vi "Data Rad For Buffer AI.vi"(8 "error In":errorcluster, 10 "Start Address":i32=1350, 11 "connection ID IN":refnum<k5>) -> (0 "error out":errorcluster, 2 "Data":dbl[](array[numeric]) format="%#.6f", 3 "connection ID OUT":refnum<k5>)   [LabVIEW 2015]
panel:
  out "concatenated string":string
  out "Array":string[](array[string])
  out "Numeric":i32
  out "bytes written1":i32
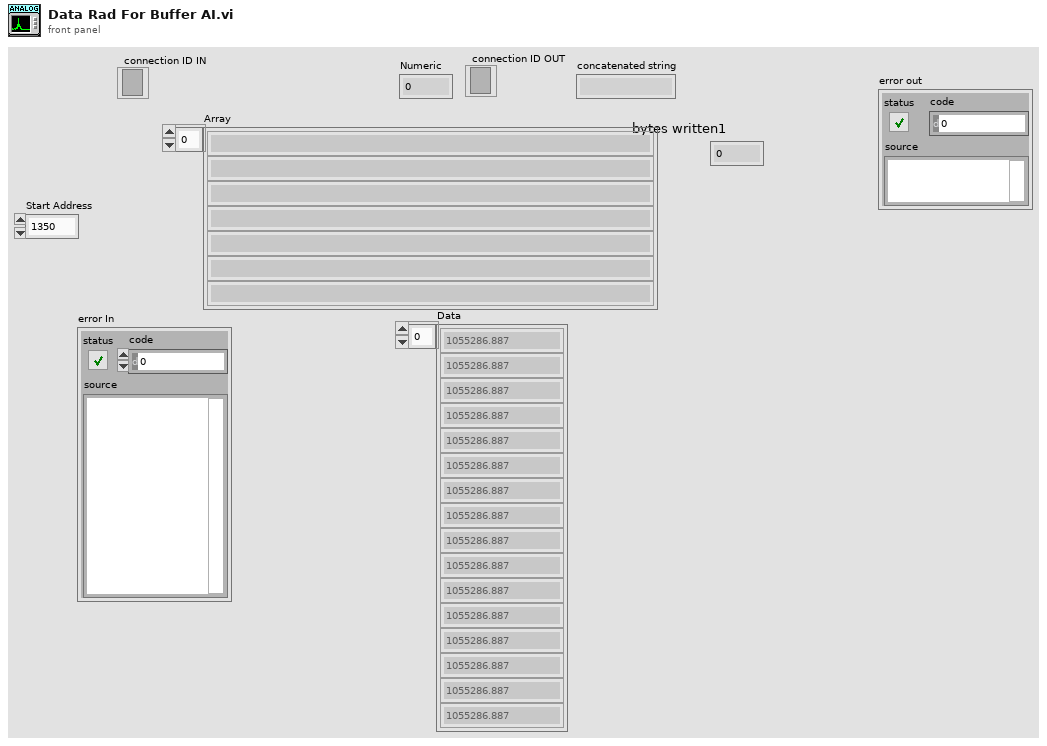
[diagram p1: front panel]
types:
  T1 = enum16{"Standard", "Buffered", "CRLF", "Immediate"}
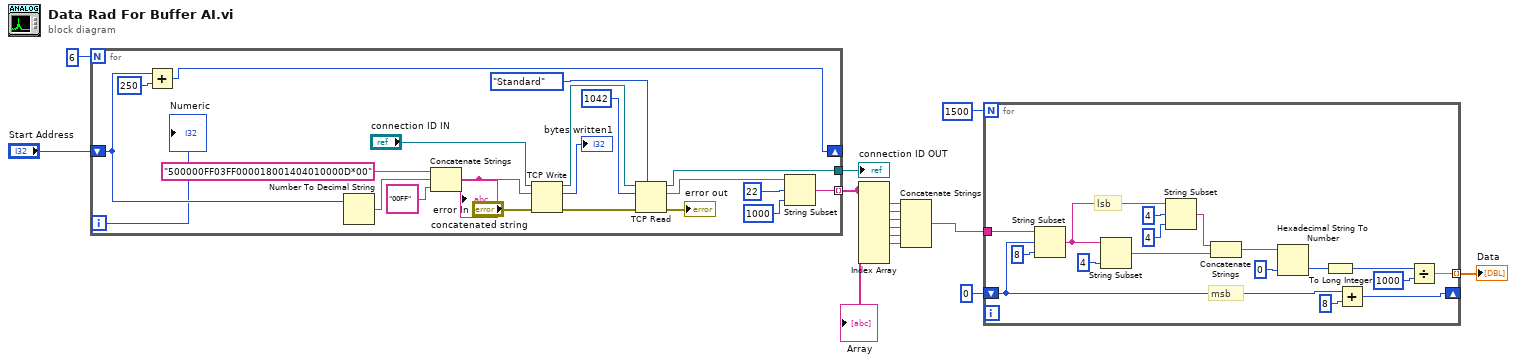
[diagram p0: block diagram]
diagram:
  n1 = for {
    N: 6 -> [_]
    tunnel: [w18] -> w9 mode=indexing
    tunnel: [w25] -> w13
    shift-right: [w22] -> _
    shift-left: "Start Address" -> [w24]
    i -> [w15]
    n2 = Add(x=w24, y=250) -> (x+y=w22:i32)
    n3 = Number To Decimal String(number=w24) -> (decimal integer string=w32:string)  [unwired: 1 in]
    n4 = Concatenate Strings("500000FF03FF000018001404010000D*00", w32, "00FF" ("String")) -> (w34:string)
    "concatenated string" <- w34
    n5 = TCP Write(connection ID="connection ID IN", data in=w34, error in (no error)="error In") -> (connection ID out=w29:refnum<k5>, bytes written=→"bytes written1":i32, error out=w28:errorcluster)  [unwired: 1 in]
    n6 = TCP Read(connection ID=w29, bytes to read=1042, error in (no error)=w28, 7:T1."Standard" ("mode (standard)")) -> (connection ID out=w25:refnum<k5>, data out=w19:string, error out=→"error out":errorcluster)  [unwired: 1 in]
    n7 = String Subset(string=w19, offset (0)=22, length (rest)=1000 ("length (rest)")) -> (substring=w18:string)
    "Numeric" <- w15
  }
  "connection ID OUT" <- w13
  "Array" <- w9
  n8 = Index Array(array=w9) -> (element #1=w7:string, element #2=w6:string, element #3=w5:string, element #4=w4:string, element #5=w2:string, element #6=w1:string)  [unwired: 8 in, 2 out]
  n9 = Concatenate Strings(w7, w6, w5, w4, w2, w1) -> (w3:string)
  n10 = for {
    N: 1500 ("Length") -> [_]
    shift-right: [w52] -> _
    shift-left: 0 -> [w49]
    tunnel: w3 -> [w50]
    tunnel: [w36] -> w10 mode=indexing
    # "lsb"
    # "msb"
    n11 = String Subset(string=w50, offset (0)=w49, length (rest)=8 ("length (rest)")) -> (substring=w44:string)
    n12 = String Subset(string=w44, length (rest)=4 ("length (rest)")) -> (substring=w42:string)  [unwired: 1 in]
    n13 = String Subset(string=w44, offset (0)=4, length (rest)=4 ("length (rest)")) -> (substring=w43:string)
    n14 = Concatenate Strings(w43, w42) -> (w41:string)
    n15 = Hexadecimal String To Number(string=w41, default (0uL)=u32 0 ("default (0 U32)")) -> (number=w37:u32)  [unwired: 1 in, 1 out]
    n16 = To Long Integer(number=w37) -> (32bit integer=w38:i32)
    n17 = Add(x=w49, y=8) -> (x+y=w52:i32)
    n18 = Divide(x=w38, y=u32 1000) -> (x/y=w36:dbl)
  }
  "Data" <- w10
